vi "ErrorLogRef Global.vi"() -> ()   [LabVIEW 2019, in "ErrorLog.lvlib" / "ErrorLog.lvclass"]
uses:
  ErrorLog.lvclass
panel:
  in  "ErrorLogRef":refnum<class "ErrorLog.lvclass">
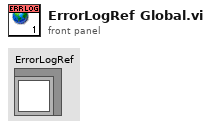
[diagram p1: front panel]
diagram:
